vi "FPGAcode_6_02_14.vi"() -> ()   [LabVIEW 2013]
uses:
  <vilib>/Platform/TimedLoop/XDataNode/timing_clust.ctl
  <vilib>/Platform/TimedLoop/XDataNode/nitl_modes.ctl
  <vilib>/Platform/TimedLoop/XDataNode/wakeup.ctl
  <vilib>/rvi/Emulation/niFpgaSctlEmulationGetInTimedLoop.vi
  <vilib>/rvi/Emulation/niFpgaEmulationReportErrorSimple.vi
  <vilib>/rvi/Emulation/niFpgaGetClockAttributes.vi
  <vilib>/rvi/Emulation/niFpgaCriticalErrorInLSC.vi
  <vilib>/rvi/eio/common/nirviEmuTemplateMethod_errors.vi
  <vilib>/Platform/TimedLoop/XDataNode/XDataNode.xnode
  <vilib>/eio/EIONode/EIONode.xnode
  <vilib>/Platform/TimedLoop/XDataNode/XDNodeRunTimeDep.lvlib
panel:
  out "Not Armed?":bool
  in  "Reset One Shot":bool
  in  "One Shot":bool
  in  "Mult1 Use":bool
  out "Filter 1 Detector 3 Correlation":i32
  in  "Filter 2 threshold":i32=1000
  out "Filter 2 Detector 3 Correlation":i32
  in  "Filter 1 threshold":i32=1000
  in  "Filter 3 threshold":i32=1000
  out "Filter 3 Detector 3 Correlation":i32
  in  "Filter 4 threshold":i32=1000
  out "Filter 4 Detector 3 Correlation":i32
  in  "Filter 5 threshold":i32
  out "Filter 5 Detector 3 Correlation":i32
  in  "Filter 6 threshold":i32
  out "Filter 6 Detector 3 Correlation":i32
  in  "Filter 7 threshold":i32
  out "Filter 7 Detector 3 Correlation":i32
  out "Plates":bool
  in  "High Charge Limit":i16
  in  "Low Charge Limit":i16
  in  "High Velocity Count":i32
  in  "Low Velocity Count":i32
  in  "High Mass Limit":i64
  in  "Low Mass Limit":i64
  in  "Mult1":fxp<+,16,7>
  out "Delay1":bool
  out "IO Module\\AI 0":i16
  out "IO Module\\AI 1":i16
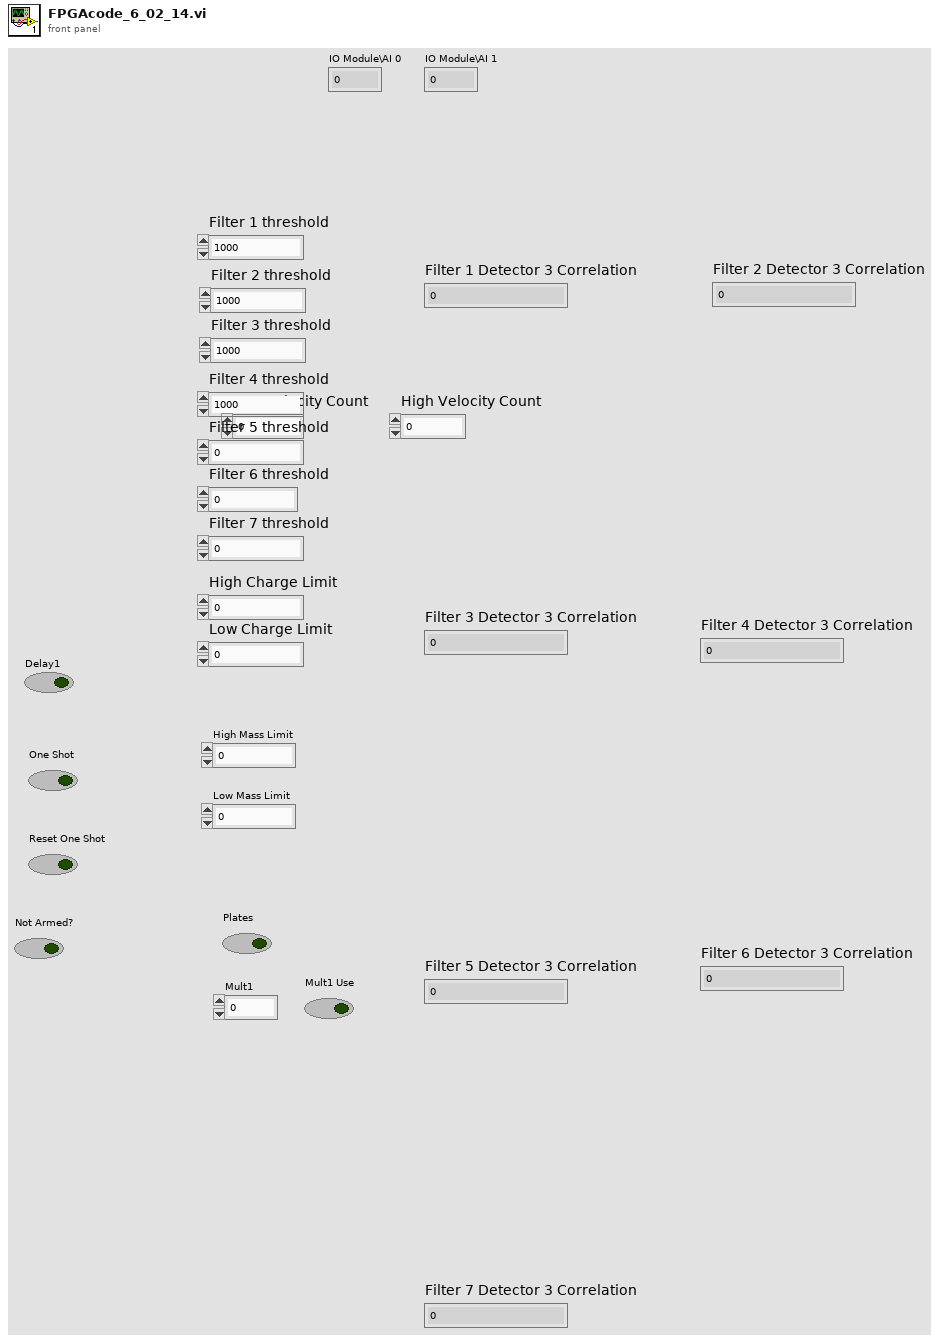
[diagram p1: front panel]
types:
  T1 = typedef "XDNodeRunTimeDep.lvlib/timing_clust.ctl" = cluster{"Expected End [f-1]":u64, "Actual End [f-1]":u64, "Finished Late? [f-1]":bool, "Expected End [i-1]":u64, "Actual End [i-1]":u64, "Finished Late? [i-1]":bool, "Expected Start [i]":u64, "Actual Start [i]":u64, "Expected Start [f]":u64, "Actual Start [f]":u64, "Source Name":string, "Structure Name":string, "Period":i64, "Deadline":i64, "Offset":i64, "Start":i64, "Priority":i32, "Timeout":i32, "Mode":T2, "Wakeup Reason":T3, "Error":errorcluster, "Source Type":string, "Secondary Source Type":string, "Global End Time":u64, "Global Start Time":u64, "Frame Duration":u64, "Iteration Duration":u64, "Assigned CPU":i32, "I/O Scan Engine Mode":u32}
  T2 = typedef "XDNodeRunTimeDep.lvlib/nitl_modes.ctl" = enum32{"No Change", "Process missed periods, maintain original phase", "Discard missed periods, maintain original phase", "Process missed periods, ignore original phase", "Discard missed periods, ignore original phase"}
  T3 = typedef "XDNodeRunTimeDep.lvlib/wakeup.ctl" = enum32{"Normal", "Aborted", "Asynchronous wakeup", "Timing source error", "Timed loop error", "Timeout"}
  T4 = cluster{"Separation cut off 1":i32, "Filter Number":i32, "Separation cut off 2":i32}
  T5 = cluster{"Old Average":i32, "New Average":i32, "Current State":u8, "Detector 1 Correlation":i32, "Detector 3 Correlation":i32, "Velocity Count":i32, "Detector Counter in":i32, "Timeout Count in":i32, "Measured Charge in":i32, "Filter Threshold":i32, "High Correlation in":i32, "Offset":i32, "Offset Average":i32, "Measured Velocity In":i32, "Mult Cluster":cluster{"Mult1":fxp<+,16,7>, "Mult1 Use?":bool}, "Final Delay Count In":u16, "Delay1 In":i32}
  T6 = cluster{"High Charge Limit":i16, "Low Charge Limit":i16, "Low Velocity Count":i32, "High Velocity Count":i32, "Low Velocity Count":i32, fxp<+,30,25>, "High Mass Limit":i64, "Low Mass Limit":i64}
  T7 = cluster{"Average Out":i32, "Next State":u8, "Velocity Count out":i32, "Detector counter out":i32, "Timeout count out":u32, "Measured Charge Out":i32, "High Correlation Out":i32, "Plates":bool, "Offset Out":i32, "Measured Velocity Out":i32, "Final Delay Count Out":u16, "Out1":bool, "Delay1":i32}
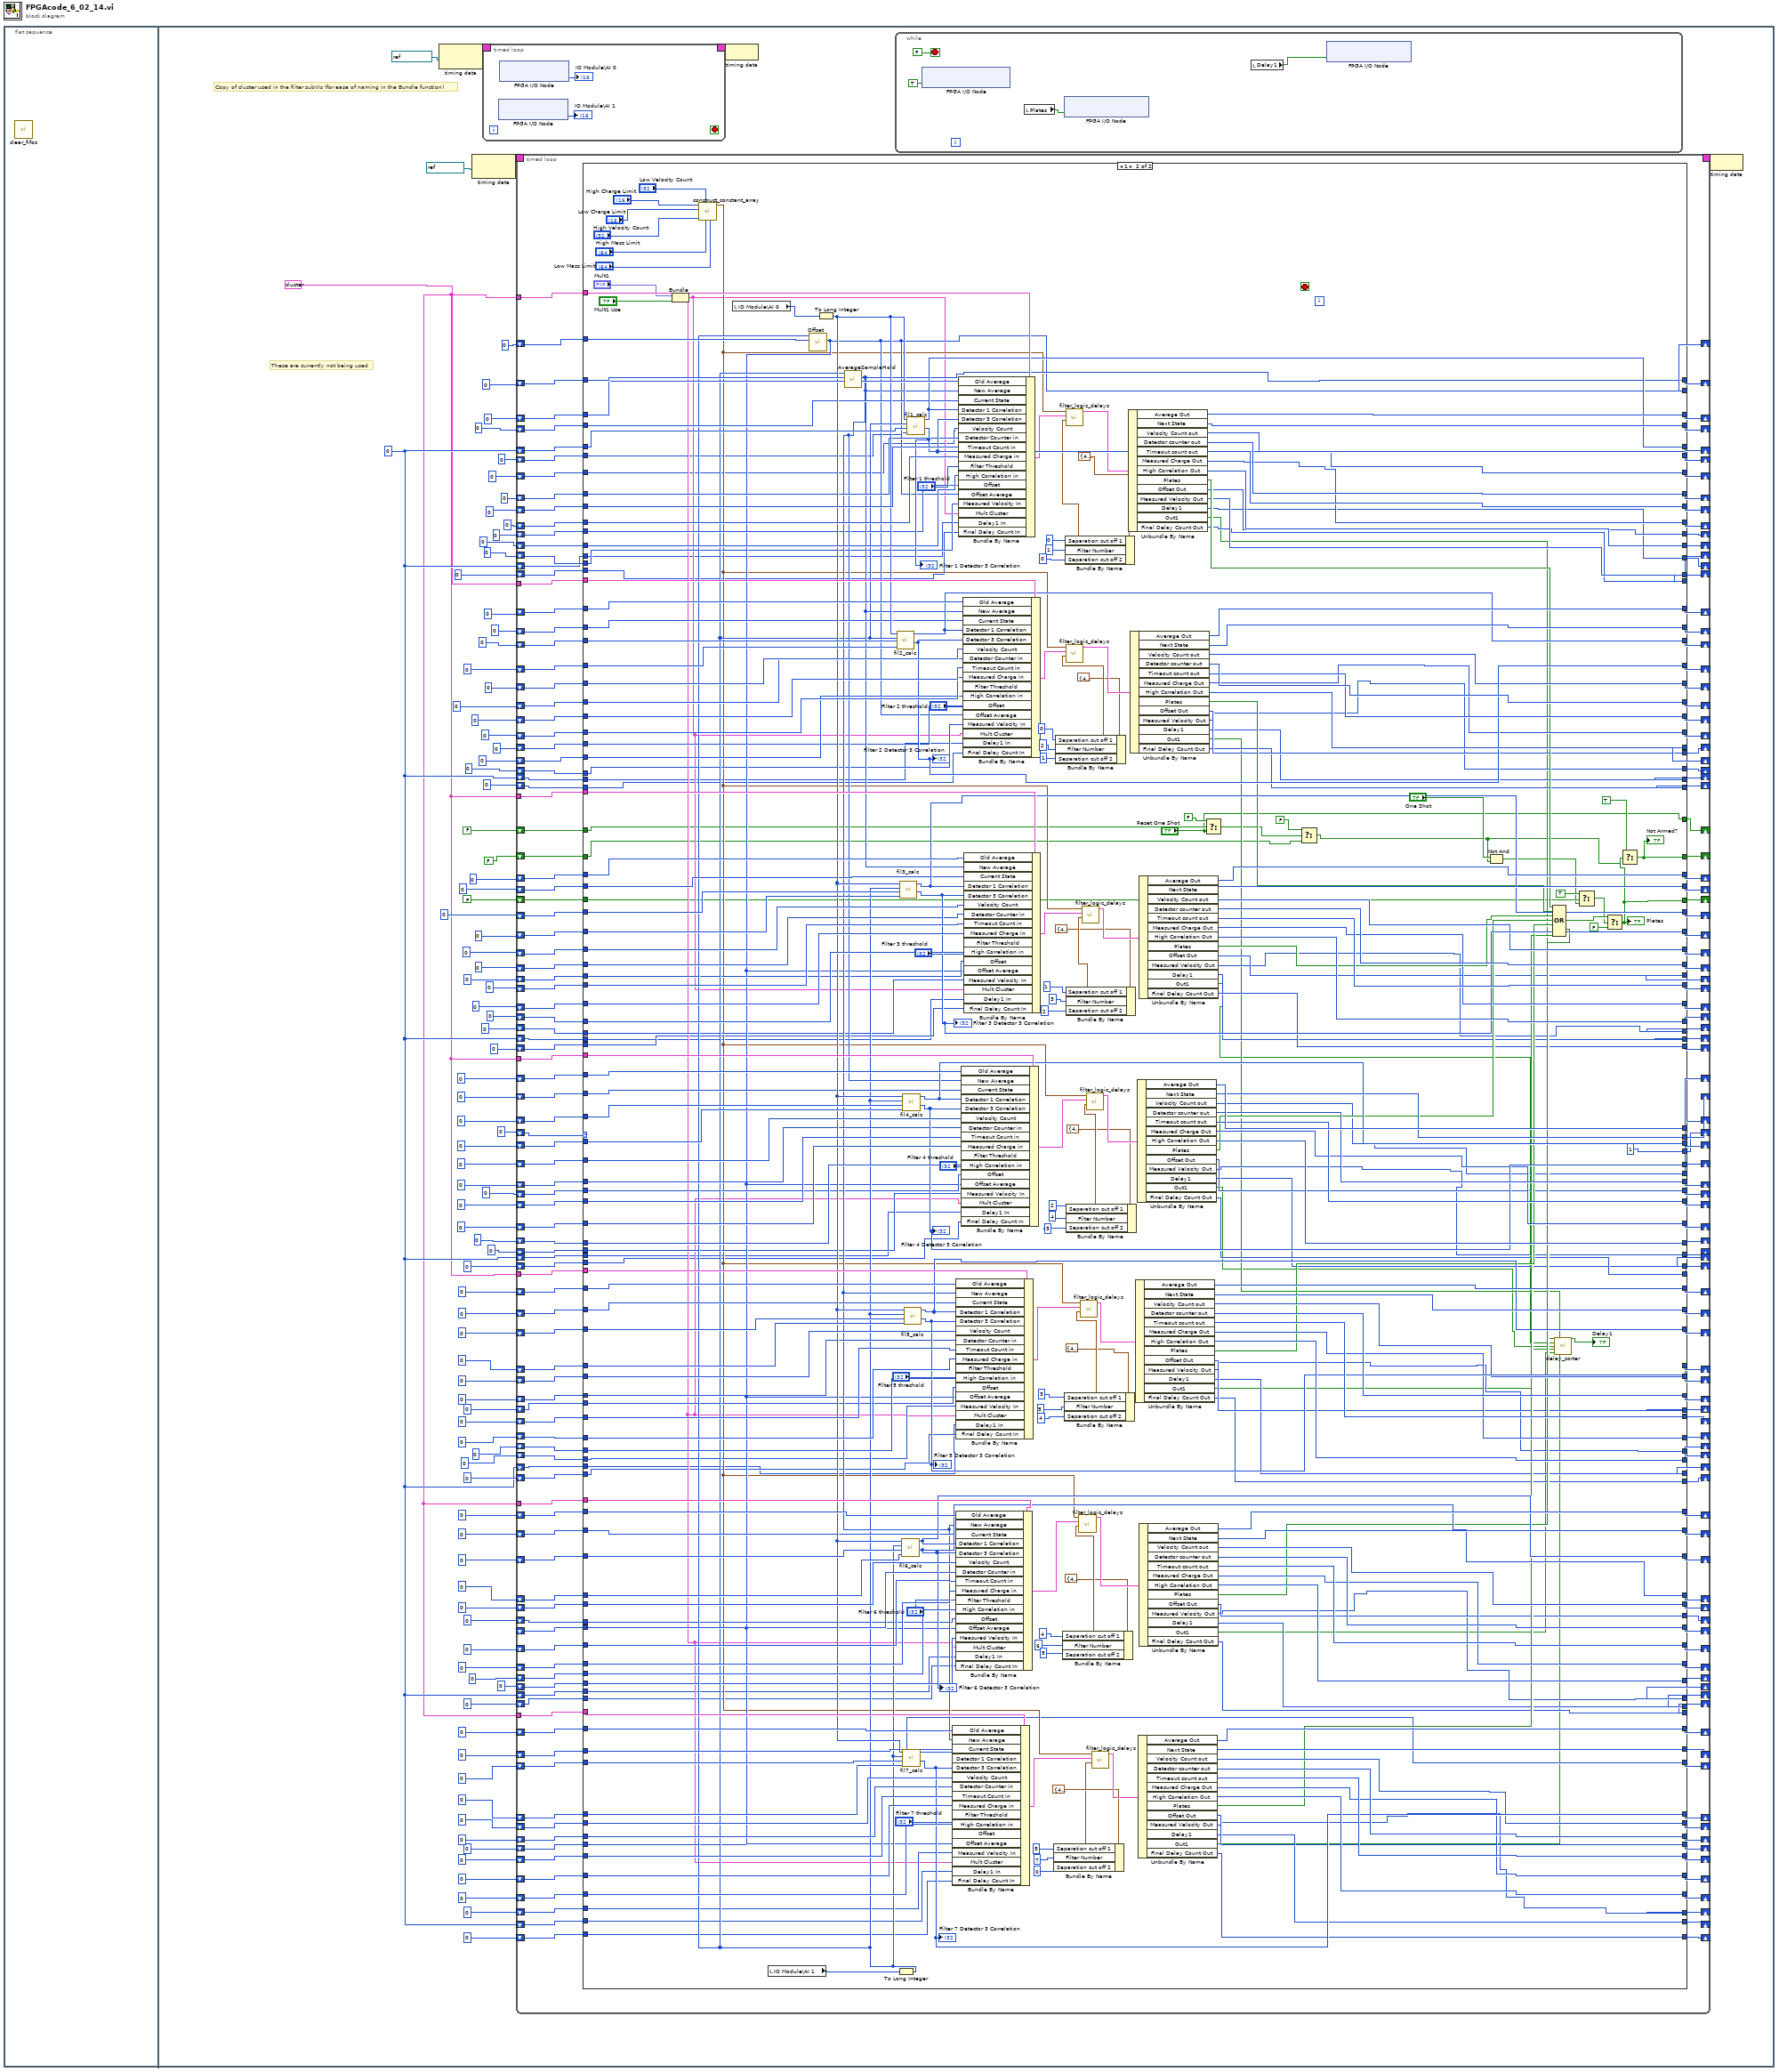
[diagram p0: block diagram]
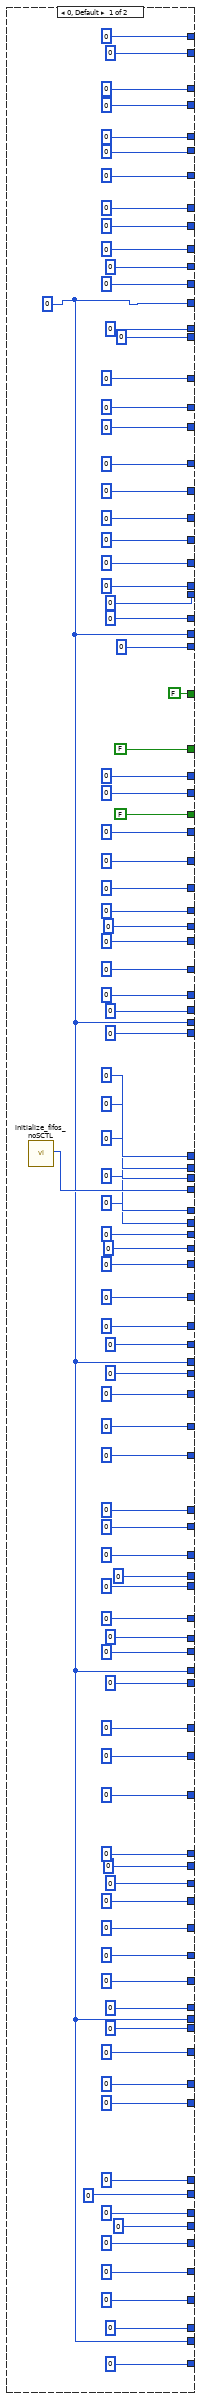
[diagram p2: hidden frame]
diagram:
  n1 = flat-sequence {
    frame #0 {
      n2 = call "clear_fifos.vi"() -> ()  [unwired: 1 in]
    }
    frame #1 {
      w2 = T5 {"Old Average"=0, "New Average"=0, "Current State"=0, "Detector 1 Correlation"=0, "Detector 3 Correlation"=0, "Velocity Count"=0, "Detector Counter in"=0, "Timeout Count in"=0, "Measured Charge in"=0, "Filter Threshold"=0, "High Correlation in"=0, "Offset"=0, "Offset Average"=0, "Measured Velocity In"=0, "Mult Cluster"={"Mult1"=0.0, "Mult1 Use?"=FALSE}, "Final Delay Count In"=0, "Delay1 In"=0} ("Variables Cluster")
      w5 = 0 ("Detector 1 Correlation Out")
      # "These are currently not being used"
      # "Copy of cluster used in the filter subVIs (for ease of naming in the Bundle function)"
      n3 = node-c288(refnum<k21> "AI Clock" ("Source Name")) -> (w32:T1)
      n4 = node-c288(refnum<k21> "26 MHz" ("Source Name")) -> (w96:T1)
      n5 = timed-loop {
        timing: w32 -> [_]
        timing-out: [_] -> w31
        stop <- _ stop-if-true
        n6 = xnode "FPGA I/O Node"() -> ("IO Module\\AI 1"=→"IO Module\\AI 1":i16)  [unwired: 1 in, 1 out]
        n7 = xnode "FPGA I/O Node"() -> ("IO Module\\AI 0"=→"IO Module\\AI 0":i16)  [unwired: 1 in, 1 out]
      }
      n8 = timed-loop {
        timing: w96 -> [_]
        timing-out: [_] -> w95
        shift-right: [w302] -> _
        shift-left: 0 ("Velocity Count out") -> [w224]
        shift-right: [w303] -> _
        shift-left: 0 ("Detector 1 Correlation out") -> [w225]
        shift-right: [w189] -> _
        shift-left: 0 ("Detector counter out") -> [w226]
        shift-right: [w220] -> _
        shift-left: 0 ("Next State") -> [w227]
        shift-right: [w188] -> _
        shift-left: 0 ("Detector 3 Correlation out") -> [w223]
        shift-right: [w301] -> _
        shift-left: 0 ("Timeout count out") -> [w222]
        shift-right: [w216] -> _
        shift-left: 0 ("Next State") -> [w219]
        shift-right: [w215] -> _
        shift-left: 0 ("Detector counter out") -> [w218]
        shift-right: [w187] -> _
        shift-left: 0 ("Detector 1 Correlation out") -> [w295]
        shift-right: [w292] -> _
        shift-left: 0 ("Velocity Count out") -> [w294]
        shift-right: [w291] -> _
        shift-left: u32 0 ("Detector 3 Correlation out") -> [w293]
        shift-right: [w286] -> _
        shift-left: 0 ("Timeout count out") -> [w287]
        shift-right: [w210] -> _
        shift-left: 0 ("Next State") -> [w213]
        shift-right: [w185] -> _
        shift-left: 0 ("Detector counter out") -> [w283]
        shift-right: [w281] -> _
        shift-left: 0 ("Detector 1 Correlation out") -> [w282]
        shift-right: [w279] -> _
        shift-left: u32 0 ("Velocity Count out") -> [w280]
        shift-right: [w184] -> _
        shift-left: 0 ("Detector 3 Correlation out") -> [w278]
        shift-right: [w277] -> _
        shift-left: 0 ("Timeout count out") -> [w212]
        shift-right: [w304] -> _
        shift-left: u8 0 ("High Correlation Out") -> [w307]
        shift-right: [w296] -> _
        shift-left: u8 0 ("High Correlation Out") -> [w297]
        shift-right: [w211] -> _
        shift-left: 0 ("High Correlation Out") -> [w214]
        shift-right: [w305] -> _
        shift-left: 0 ("Measured Charge Out") -> [w308]
        shift-right: [w298] -> _
        shift-left: 0 ("Measured Charge Out") -> [w299]
        shift-right: [w285] -> _
        shift-left: u8 0 ("Measured Charge Out") -> [w284]
        shift-right: [w175] -> _
        shift-left: 0 ("Output New Average") -> [w309]
        shift-right: [w221] -> _
        shift-left: w5 -> [w228]
        tunnel: w2 -> [w306]
        shift-right: [w186] -> _
        shift-left: 0 ("High Sample Out") -> [w289]
        shift-right: [w290] -> _
        shift-left: 0 ("High Correlation Out") -> [w217]
        tunnel: w2 -> [w300]
        tunnel: w2 -> [w288]
        shift-right: [w276] -> _
        shift-left: 0 ("Average Out") -> [w275]
        shift-right: [w274] -> _
        shift-left: u8 0 ("Next State") -> [w273]
        shift-right: [w206] -> _
        shift-left: 0 ("Detector 1 Correlation out") -> [w208]
        shift-right: [w205] -> _
        shift-left: 0 ("Detector 3 Correlation out") -> [w207]
        shift-right: [w183] -> _
        shift-left: 0 ("Velocity Count out") -> [w272]
        shift-right: [w271] -> _
        shift-left: 0 ("Detector counter out") -> [w270]
        shift-right: [w269] -> _
        shift-left: u32 0 ("Timeout count out") -> [w268]
        shift-right: [w182] -> _
        shift-left: 0 ("Measured Charge Out") -> [w267]
        shift-right: [w266] -> _
        shift-left: 0 ("High Correlation Out") -> [w209]
        tunnel: w2 -> [w265]
        shift-right: [w263] -> _
        shift-left: 0 ("Average Out") -> [w262]
        shift-right: [w261] -> _
        shift-left: u8 0 ("Next State") -> [w260]
        shift-right: [w201] -> _
        shift-left: 0 ("Detector 1 Correlation out") -> [w204]
        shift-right: [w200] -> _
        shift-left: 0 ("Detector 3 Correlation out") -> [w203]
        shift-right: [w181] -> _
        shift-left: 0 ("Velocity Count out") -> [w259]
        shift-right: [w258] -> _
        shift-left: 0 ("Detector counter out") -> [w257]
        shift-right: [w256] -> _
        shift-left: u32 0 ("Timeout count out") -> [w255]
        shift-right: [w180] -> _
        shift-left: 0 ("Measured Charge Out") -> [w254]
        shift-right: [w253] -> _
        shift-left: 0 ("High Correlation Out") -> [w202]
        tunnel: w2 -> [w264]
        shift-right: [w251] -> _
        shift-left: 0 ("Average Out") -> [w249]
        shift-right: [w250] -> _
        shift-left: u8 0 ("Next State") -> [w246]
        shift-right: [w196] -> _
        shift-left: 0 ("Detector 1 Correlation out") -> [w199]
        shift-right: [w195] -> _
        shift-left: 0 ("Detector 3 Correlation out") -> [w198]
        shift-right: [w178] -> _
        shift-left: 0 ("Velocity Count out") -> [w248]
        shift-right: [w245] -> _
        shift-left: _ -> [w247]
        shift-right: [w244] -> _
        shift-left: u32 0 ("Timeout count out") -> [w243]
        shift-right: [w179] -> _
        shift-left: 0 ("Measured Charge Out") -> [w242]
        shift-right: [w241] -> _
        shift-left: 0 ("High Correlation Out") -> [w197]
        tunnel: w2 -> [w252]
        shift-right: [w239] -> _
        shift-left: 0 ("Average Out") -> [w238]
        shift-right: [w237] -> _
        shift-left: u8 0 ("Next State") -> [w229]
        shift-right: [w191] -> _
        shift-left: 0 ("Detector 1 Correlation out") -> [w194]
        shift-right: [w190] -> _
        shift-left: 0 ("Detector 3 Correlation out") -> [w193]
        shift-right: [w177] -> _
        shift-left: 0 ("Velocity Count out") -> [w236]
        shift-right: [w235] -> _
        shift-left: 0 ("Detector counter out") -> [w234]
        shift-right: [w233] -> _
        shift-left: u32 0 ("Timeout count out") -> [w232]
        shift-right: [w176] -> _
        shift-left: 0 ("Measured Charge Out") -> [w231]
        shift-right: [w230] -> _
        shift-left: 0 ("High Correlation Out") -> [w192]
        tunnel: w2 -> [w240]
        shift-right: [w173] -> _
        shift-left: i16 0 -> [w174]
        shift-right: [w171] -> _
        shift-left: 0 -> [w172]
        shift-right: [w170] -> _
        shift-left: 0 -> [w167]
        shift-right: [w168] -> _
        shift-left: 0 -> [w169]
        shift-right: [w165] -> _
        shift-left: 0 ("Offset Out") -> [w166]
        shift-right: [w164] -> _
        shift-left: 0 ("Offset Out") -> [w163]
        shift-right: [w162] -> _
        shift-left: 0 ("Offset Out") -> [w161]
        shift-right: [w160] -> _
        shift-left: 0 ("Offset Out") -> [w159]
        shift-right: [w158] -> _
        shift-left: 0 ("Offset Out") -> [w157]
        shift-right: [w155] -> _
        shift-left: 0 -> [w156]
        shift-right: [w154] -> _
        shift-left: 0 -> [w143]
        shift-right: [w153] -> _
        shift-left: 0 -> [w144]
        shift-right: [w152] -> _
        shift-left: 0 -> [w145]
        shift-right: [w151] -> _
        shift-left: 0 -> [w146]
        shift-right: [w150] -> _
        shift-left: 0 -> [w147]
        shift-right: [w149] -> _
        shift-left: 0 ("Measured Velocity Out") -> [w148]
        shift-right: [w142] -> _
        shift-left: w5 -> [w140]
        shift-right: [w141] -> _
        shift-left: u32 0 ("Final Delay Count Out") -> [w139]
        shift-right: [w138] -> _
        shift-left: w5 -> [w136]
        shift-right: [w137] -> _
        shift-left: u32 0 ("Final Delay Count Out") -> [w135]
        shift-right: [w134] -> _
        shift-left: w5 -> [w132]
        shift-right: [w133] -> _
        shift-left: u32 0 ("Final Delay Count Out") -> [w131]
        shift-right: [w130] -> _
        shift-left: w5 -> [w128]
        shift-right: [w129] -> _
        shift-left: u32 0 ("Final Delay Count Out") -> [w127]
        shift-right: [w126] -> _
        shift-left: w5 -> [w124]
        shift-right: [w125] -> _
        shift-left: u32 0 ("Final Delay Count Out") -> [w123]
        shift-right: [w122] -> _
        shift-left: w5 -> [w120]
        shift-right: [w121] -> _
        shift-left: u32 0 ("Final Delay Count Out") -> [w119]
        shift-right: [w118] -> _
        shift-left: w5 -> [w116]
        shift-right: [w117] -> _
        shift-left: u32 0 ("Final Delay Count Out") -> [w115]
        shift-right: [w113] -> _
        shift-left: FALSE -> [w114]
        shift-right: [w112] -> _
        shift-left: FALSE ("f") -> [w111]
        shift-right: [w110] -> _
        shift-left: FALSE ("Reset One Shot") -> [w109]
        stop <- _ stop-if-true
        n9 = case shown="1" w174 {
          tunnel: w309 -> [_ w696]
          tunnel: w308 -> [_ w695]
          tunnel: w307 -> [_ w530]
          tunnel: w306 -> [_ w694]
          tunnel: [0 ("Average Out") w693] -> w305
          tunnel: [u16 0 ("Next State") w692] -> w304
          tunnel: [0 ("Detector counter out") w691] -> w303
          tunnel: [u32 0 ("Timeout count out") w690] -> w302
          tunnel: [0 ("High Correlation Out") w689] -> w301
          tunnel: w300 -> [_ w688]
          tunnel: w299 -> [_ w687]
          tunnel: [0 ("Average Out") w686] -> w298
          tunnel: w297 -> [_ w529]
          tunnel: [u16 0 ("Next State") w685] -> w296
          tunnel: w295 -> [_ w684]
          tunnel: w294 -> [_ w522]
          tunnel: w293 -> [_ w683]
          tunnel: [0 ("Detector counter out") w682] -> w292
          tunnel: [u32 0 ("Timeout count out") w681] -> w291
          tunnel: [0 ("High Correlation Out") w680] -> w290
          tunnel: w289 -> [_ w679]
          tunnel: w288 -> [_ w678]
          tunnel: w287 -> [_ w677]
          tunnel: [0 ("Average Out") w676] -> w286
          tunnel: [u16 0 ("Next State") w675] -> w285
          tunnel: w284 -> [_ w528]
          tunnel: w283 -> [_ w674]
          tunnel: w282 -> [_ w521]
          tunnel: [0 ("Detector counter out") w673] -> w281
          tunnel: w280 -> [_ w672]
          tunnel: [u32 0 ("Timeout count out") w671] -> w279
          tunnel: w278 -> [_ w670]
          tunnel: [0 ("High Correlation Out") w669] -> w277
          tunnel: [0 ("Average Out") w668] -> w276
          tunnel: w275 -> [_ w667]
          tunnel: [u16 0 ("Next State") w666] -> w274
          tunnel: w273 -> [_ w527]
          tunnel: w272 -> [_ w665]
          tunnel: [0 ("Detector counter out") w664] -> w271
          tunnel: w270 -> [_ w520]
          tunnel: [u32 0 ("Timeout count out") w663] -> w269
          tunnel: w268 -> [_ w662]
          tunnel: w267 -> [_ w661]
          tunnel: [0 ("High Correlation Out") w660] -> w266
          tunnel: w265 -> [_ w659]
          tunnel: w264 -> [_ w658]
          tunnel: [0 ("Average Out") w657] -> w263
          tunnel: w262 -> [_ w656]
          tunnel: [u16 0 ("Next State") w655] -> w261
          tunnel: w260 -> [_ w526]
          tunnel: w259 -> [_ w654]
          tunnel: [0 ("Detector counter out") w653] -> w258
          tunnel: w257 -> [_ w519]
          tunnel: [u32 0 ("Timeout count out") w652] -> w256
          tunnel: w255 -> [_ w651]
          tunnel: w254 -> [_ w650]
          tunnel: [0 ("High Correlation Out") w649] -> w253
          tunnel: w252 -> [_ w648]
          tunnel: [0 ("Average Out") w647] -> w251
          tunnel: [u16 0 ("Next State") w646] -> w250
          tunnel: w249 -> [_ w645]
          tunnel: w248 -> [_ w644]
          tunnel: w247 -> [_ w518]
          tunnel: w246 -> [_ w525]
          tunnel: [0 ("Detector counter out") w643] -> w245
          tunnel: [u32 0 ("Timeout count out") w642] -> w244
          tunnel: w243 -> [_ w641]
          tunnel: w242 -> [_ w640]
          tunnel: [0 ("High Correlation Out") w639] -> w241
          tunnel: w240 -> [_ w638]
          tunnel: [0 ("Average Out") w637] -> w239
          tunnel: w238 -> [_ w636]
          tunnel: [u16 0 ("Next State") w635] -> w237
          tunnel: w236 -> [_ w634]
          tunnel: [0 ("Detector counter out") w633] -> w235
          tunnel: w234 -> [_ w517]
          tunnel: [u32 0 ("Timeout count out") w632] -> w233
          tunnel: w232 -> [_ w631]
          tunnel: w231 -> [_ w630]
          tunnel: [0 ("High Correlation Out") w629] -> w230
          tunnel: w229 -> [_ w524]
          tunnel: w228 -> [_ w628]
          tunnel: w227 -> [_ w423]
          tunnel: w226 -> [_ w424]
          tunnel: w225 -> [_ w523]
          tunnel: w224 -> [_ w627]
          tunnel: w223 -> [_ w626]
          tunnel: w222 -> [_ w625]
          tunnel: [0 ("Detector 1 Correlation Out") w624] -> w221
          tunnel: [0 ("Detector 3 Correlation Out") w623] -> w220
          tunnel: w219 -> [_ w622]
          tunnel: w218 -> [_ w621]
          tunnel: w217 -> [_ w620]
          tunnel: [0 ("Detector 1 Correlation Out") w619] -> w216
          tunnel: [0 ("Detector 3 Correlation Out") w618] -> w215
          tunnel: w214 -> [_ w617]
          tunnel: w213 -> [_ w616]
          tunnel: w212 -> [_ w615]
          tunnel: [0 ("Detector 1 Correlation Out") w614] -> w211
          tunnel: [0 ("Detector 3 Correlation Out") w613] -> w210
          tunnel: w209 -> [_ w612]
          tunnel: w208 -> [_ w611]
          tunnel: w207 -> [_ w610]
          tunnel: [0 ("Detector 1 Correlation Out") w609] -> w206
          tunnel: [0 ("Detector 3 Correlation Out") w608] -> w205
          tunnel: w204 -> [_ w607]
          tunnel: w203 -> [_ w606]
          tunnel: w202 -> [_ w605]
          tunnel: [0 ("Detector 1 Correlation Out") w604] -> w201
          tunnel: [0 ("Detector 3 Correlation Out") w603] -> w200
          tunnel: w199 -> [_ w602]
          tunnel: w198 -> [_ w601]
          tunnel: w197 -> [_ w600]
          tunnel: [0 ("Detector 1 Correlation Out") w599] -> w196
          tunnel: [0 ("Detector 3 Correlation Out") w598] -> w195
          tunnel: w194 -> [_ w597]
          tunnel: w193 -> [_ w596]
          tunnel: w192 -> [_ w595]
          tunnel: [0 ("Detector 1 Correlation Out") w460] -> w191
          tunnel: [0 ("Detector 3 Correlation Out") w594] -> w190
          tunnel: [0 ("Velocity Count out") w593] -> w189
          tunnel: [0 ("Measured Charge Out") w592] -> w188
          tunnel: [0 ("Velocity Count out") w591] -> w187
          tunnel: [0 ("Measured Charge Out") w590] -> w186
          tunnel: [0 ("Velocity Count out") w589] -> w185
          tunnel: [0 ("Measured Charge Out") w588] -> w184
          tunnel: [0 ("Velocity Count out") w516] -> w183
          tunnel: [0 ("Measured Charge Out") w587] -> w182
          tunnel: [0 ("Velocity Count out") w586] -> w181
          tunnel: [0 ("Measured Charge Out") w585] -> w180
          tunnel: [0 ("Measured Charge Out") w584] -> w179
          tunnel: [0 ("Velocity Count out") w583] -> w178
          tunnel: [0 ("Velocity Count out") w582] -> w177
          tunnel: [0 ("Measured Charge Out") w581] -> w176
          tunnel: [0 ("Output New Average") w515] -> w175
          tunnel: [w400 i16 1 ("Output State")] -> w173
          tunnel: w172 -> [_ w512]
          tunnel: [0 ("Offset Out") w511] -> w171
          tunnel: [0 ("Offset Out") w510] -> w170
          tunnel: w169 -> [_ w509]
          tunnel: [0 ("Output New Average") w498] -> w168
          tunnel: w167 -> [_ w507]
          tunnel: w166 -> [_ w506]
          tunnel: [0 ("Offset Out") w505] -> w165
          tunnel: [0 ("Offset Out") w504] -> w164
          tunnel: w163 -> [_ w503]
          tunnel: [0 ("Offset Out") w502] -> w162
          tunnel: w161 -> [_ w501]
          tunnel: [0 ("Offset Out") w500] -> w160
          tunnel: w159 -> [_ w499]
          tunnel: [0 ("Offset Out") w497] -> w158
          tunnel: w157 -> [_ w496]
          tunnel: w156 -> [_ w491]
          tunnel: [0 ("Measured Velocity Out") w484] -> w155
          tunnel: [0 ("Measured Velocity Out") w483] -> w154
          tunnel: [0 ("Measured Velocity Out") w482] -> w153
          tunnel: [0 ("Measured Velocity Out") w481] -> w152
          tunnel: [0 ("Measured Velocity Out") w480] -> w151
          tunnel: [0 ("Measured Velocity Out") w479] -> w150
          tunnel: [0 ("Measured Velocity Out") w478] -> w149
          tunnel: w148 -> [_ w490]
          tunnel: w147 -> [_ w489]
          tunnel: w146 -> [_ w488]
          tunnel: w145 -> [_ w487]
          tunnel: w144 -> [_ w486]
          tunnel: w143 -> [_ w485]
          tunnel: [w313 w455] -> w142
          tunnel: [u32 0 ("Final Delay Count Out") w473] -> w141
          tunnel: w140 -> [_ w472]
          tunnel: w139 -> [_ w471]
          tunnel: [w313 w470] -> w138
          tunnel: [u32 0 ("Final Delay Count Out") w469] -> w137
          tunnel: w136 -> [_ w468]
          tunnel: w135 -> [_ w467]
          tunnel: [w313 w453] -> w134
          tunnel: [u32 0 ("Final Delay Count Out") w466] -> w133
          tunnel: w132 -> [_ w446]
          tunnel: w131 -> [_ w465]
          tunnel: [w313 w452] -> w130
          tunnel: [u32 0 ("Final Delay Count Out") w464] -> w129
          tunnel: w128 -> [_ w445]
          tunnel: w127 -> [_ w463]
          tunnel: [w313 w451] -> w126
          tunnel: [u32 0 ("Final Delay Count Out") w462] -> w125
          tunnel: w124 -> [_ w444]
          tunnel: w123 -> [_ w461]
          tunnel: [w313 w450] -> w122
          tunnel: [u32 0 ("Final Delay Count Out") w459] -> w121
          tunnel: w120 -> [_ w443]
          tunnel: w119 -> [_ w458]
          tunnel: [w313 w449] -> w118
          tunnel: [u32 0 ("Final Delay Count Out") w457] -> w117
          tunnel: w116 -> [_ w442]
          tunnel: w115 -> [_ w456]
          tunnel: w114 -> [_ w408]
          tunnel: [FALSE ("t") w406] -> w113
          tunnel: [FALSE ("f") w420] -> w112
          tunnel: w111 -> [_ w419]
          tunnel: [FALSE ("Reset One Shot") "Reset One Shot"] -> w110
          tunnel: w109 -> [_ w404]
          frame 0, Default {
            w313 = 0
            n10 = call "initialize_fifos_noSCTL.vi"() -> ("Output State"=w400:i16)  [unwired: 11 in]
          }
          frame 1 {
            n11 = Bundle("Mult1"="Mult1", "Mult1 Use"="Mult1 Use") -> (w474:cluster{"Mult1":fxp<+,16,7>, "Mult1 Use":bool})  [unwired: 1 in]
            n12 = call "construct_constant_array.vi"("Low Mass Limit"="Low Mass Limit", "High Mass Limit"="High Mass Limit", "Low Velocity Count"="Low Velocity Count", "High Velocity Count"="High Velocity Count", "Low Charge Limit"="Low Charge Limit", "High Charge Limit"="High Charge Limit") -> ("constants cluster"=w475:T6)  [unwired: 5 in]
            n13 = local read "IO Module\\AI 0"() -> (w514:i16)
            n14 = local read "IO Module\\AI 1"() -> (w513:i16)
            n15 = To Long Integer(number=w514) -> (32bit integer=w539:i32)
            n16 = To Long Integer(number=w513) -> (32bit integer=w508:i32)
            n17 = call "Offset.vi"("Previous Average"=w509, "Input Value"=w508) -> ("Output New Average"=w498:i32)  [unwired: 7 in]
            n18 = call "AverageSampleHold.vi"("Previous Average"=w696, "Input Value"=w508) -> ("Output New Average"=w515:i32)  [unwired: 7 in]
            n19 = call "fil2_calc.vi"("Detector 3 Correlation In"=w621, "Detector 1 Correlation In"=w622, "AI1"=w508, "AI0"=w539) -> ("Detector 3 Correlation Out"=w618:i32, "Detector 1 Correlation Out"=w619:i32)  [unwired: 4 in]
            "Filter 2 Detector 3 Correlation" <- w618
            n20 = call "fil3_calc.vi"("Detector 3 Correlation In"=w616, "Detector 1 Correlation In"=w617, "AI1"=w508, "AI0"=w539) -> ("Detector 3 Correlation Out"=w613:i32, "Detector 1 Correlation Out"=w614:i32)  [unwired: 4 in]
            "Filter 3 Detector 3 Correlation" <- w613
            n21 = call "fil6_calc.vi"("Detector 3 Correlation In"=w601, "Detector 1 Correlation In"=w602, "AI1"=w508, "AI0"=w539) -> ("Detector 3 Correlation Out"=w598:i32, "Detector 1 Correlation Out"=w599:i32)  [unwired: 4 in]
            "Filter 6 Detector 3 Correlation" <- w598
            n22 = call "fil4_calc.vi"("Detector 3 Correlation In"=w610, "Detector 1 Correlation In"=w611, "AI1"=w508, "AI0"=w539) -> ("Detector 3 Correlation Out"=w608:i32, "Detector 1 Correlation Out"=w609:i32)  [unwired: 4 in]
            "Filter 4 Detector 3 Correlation" <- w608
            n23 = call "fil7_calc.vi"("Detector 3 Correlation In"=w596, "Detector 1 Correlation In"=w597, "AI1"=w508, "AI0"=w539) -> ("Detector 3 Correlation Out"=w594:i32, "Detector 1 Correlation Out"=w460:i32)  [unwired: 4 in]
            "Filter 7 Detector 3 Correlation" <- w594
            n24 = call "fil5_calc.vi"("Detector 3 Correlation In"=w606, "Detector 1 Correlation In"=w607, "AI1"=w508, "AI0"=w539) -> ("Detector 3 Correlation Out"=w603:i32, "Detector 1 Correlation Out"=w604:i32)  [unwired: 4 in]
            "Filter 5 Detector 3 Correlation" <- w603
            n25 = call "fil1_calc.vi"("Detector 3 Correlation In"=w423, "Detector 1 Correlation In"=w628, "AI1"=w508, "AI0"=w539) -> ("Detector 3 Correlation Out"=w623:i32, "Detector 1 Correlation Out"=w624:i32)  [unwired: 4 in]
            "Filter 1 Detector 3 Correlation" <- w623
            n26 = Bundle By Name(cluster=w638, "Old Average"=w636, "New Average"=w515, "Current State"=w524, "Detector 1 Correlation"=w460, "Detector 3 Correlation"=w594, "Velocity Count"=w634, "Detector Counter in"=w517, "Timeout Count in"=w631, "Measured Charge in"=w630, "Filter Threshold"="Filter 7 threshold", "High Correlation in"=w595, "Offset"=w496, "Offset Average"=w498, "Measured Velocity In"=w490, "Mult Cluster"=w474, "Delay1 In"=w442, "Final Delay Count In"=w456) -> (w409:T5)
            n27 = Bundle By Name(cluster=w648, "Old Average"=w645, "New Average"=w515, "Current State"=w525, "Detector 1 Correlation"=w599, "Detector 3 Correlation"=w598, "Velocity Count"=w644, "Detector Counter in"=w518, "Timeout Count in"=w641, "Measured Charge in"=w640, "Filter Threshold"="Filter 6 threshold", "High Correlation in"=w600, "Offset"=w499, "Offset Average"=w498, "Measured Velocity In"=w489, "Mult Cluster"=w474, "Delay1 In"=w443, "Final Delay Count In"=w458) -> (w410:T5)
            n28 = Bundle By Name(cluster=w658, "Old Average"=w656, "New Average"=w515, "Current State"=w526, "Detector 1 Correlation"=w604, "Detector 3 Correlation"=w603, "Velocity Count"=w654, "Detector Counter in"=w519, "Timeout Count in"=w651, "Measured Charge in"=w650, "Filter Threshold"="Filter 5 threshold", "High Correlation in"=w605, "Offset"=w501, "Offset Average"=w498, "Measured Velocity In"=w488, "Mult Cluster"=w474, "Delay1 In"=w444, "Final Delay Count In"=w461) -> (w411:T5)
            n29 = Bundle By Name(cluster=w694, "Old Average"=w695, "New Average"=w515, "Current State"=w530, "Detector 1 Correlation"=w624, "Detector 3 Correlation"=w623, "Velocity Count"=w424, "Detector Counter in"=w523, "Timeout Count in"=w627, "Measured Charge in"=w626, "Filter Threshold"="Filter 1 threshold", "High Correlation in"=w625, "Offset"=w512, "Offset Average"=w498, "Measured Velocity In"=w491, "Mult Cluster"=w474, "Delay1 In"=w472, "Final Delay Count In"=w471) -> (w415:T5)
            n30 = Bundle By Name(cluster=w659, "Old Average"=w667, "New Average"=w515, "Current State"=w527, "Detector 1 Correlation"=w609, "Detector 3 Correlation"=w608, "Velocity Count"=w665, "Detector Counter in"=w520, "Timeout Count in"=w662, "Measured Charge in"=w661, "Filter Threshold"="Filter 4 threshold", "High Correlation in"=w612, "Offset"=w503, "Offset Average"=w498, "Measured Velocity In"=w487, "Mult Cluster"=w474, "Delay1 In"=w445, "Final Delay Count In"=w463) -> (w412:T5)
            n31 = Bundle By Name(cluster=w688, "Old Average"=w687, "New Average"=w515, "Current State"=w529, "Detector 1 Correlation"=w619, "Detector 3 Correlation"=w618, "Velocity Count"=w684, "Detector Counter in"=w522, "Timeout Count in"=w683, "Measured Charge in"=w679, "Filter Threshold"="Filter 2 threshold", "High Correlation in"=w620, "Offset"=w507, "Offset Average"=w498, "Measured Velocity In"=w485, "Mult Cluster"=w474, "Delay1 In"=w468, "Final Delay Count In"=w467) -> (w414:T5)
            n32 = Bundle By Name(cluster=w678, "Old Average"=w677, "New Average"=w515, "Current State"=w528, "Detector 1 Correlation"=w614, "Detector 3 Correlation"=w613, "Velocity Count"=w674, "Detector Counter in"=w521, "Timeout Count in"=w672, "Measured Charge in"=w670, "Filter Threshold"="Filter 3 threshold", "High Correlation in"=w615, "Offset"=w506, "Offset Average"=w498, "Measured Velocity In"=w486, "Mult Cluster"=w474, "Delay1 In"=w446, "Final Delay Count In"=w465) -> (w413:T5)
            n33 = Bundle By Name(cluster=T4 {"Separation cut off 1"=4, "Filter Number"=5, "Separation cut off 2"=6} ("Filter Specific Constants"), "Separation cut off 1"=5, "Filter Number"=7, "Separation cut off 2"=0) -> (w427:T4)
            n34 = Bundle By Name(cluster=T4 {"Separation cut off 1"=4, "Filter Number"=5, "Separation cut off 2"=6} ("Filter Specific Constants"), "Separation cut off 1"=0, "Filter Number"=2, "Separation cut off 2"=1) -> (w572:T4)
            n35 = Bundle By Name(cluster=T4 {"Separation cut off 1"=4, "Filter Number"=5, "Separation cut off 2"=6} ("Filter Specific Constants"), "Separation cut off 1"=4, "Filter Number"=6, "Separation cut off 2"=5) -> (w562:T4)
            n36 = Bundle By Name(cluster=T4 {"Separation cut off 1"=4, "Filter Number"=5, "Separation cut off 2"=6} ("Filter Specific Constants"), "Separation cut off 1"=3, "Filter Number"=5, "Separation cut off 2"=4) -> (w564:T4)
            n37 = Bundle By Name(cluster=T4 {"Separation cut off 1"=4, "Filter Number"=5, "Separation cut off 2"=6} ("Filter Specific Constants"), "Separation cut off 1"=0, "Filter Number"=1, "Separation cut off 2"=0) -> (w570:T4)
            n38 = call "filter_logic_delays.vi"("Filter Specific Constants"=w570, "Variables Cluster"=w415, "controls cluster"=w475) -> ("Output Cluster"=w569:T7)  [unwired: 8 in]
            n39 = call "filter_logic_delays.vi"("Filter Specific Constants"=w572, "Variables Cluster"=w414, "controls cluster"=w475) -> ("Output Cluster"=w579:T7)  [unwired: 8 in]
            n40 = Bundle By Name(cluster=T4 {"Separation cut off 1"=4, "Filter Number"=5, "Separation cut off 2"=6} ("Filter Specific Constants"), "Separation cut off 1"=1, "Filter Number"=3, "Separation cut off 2"=2) -> (w568:T4)
            n41 = Bundle By Name(cluster=T4 {"Separation cut off 1"=4, "Filter Number"=5, "Separation cut off 2"=6} ("Filter Specific Constants"), "Separation cut off 1"=2, "Filter Number"=4, "Separation cut off 2"=3) -> (w566:T4)
            n42 = call "filter_logic_delays.vi"("Filter Specific Constants"=w562, "Variables Cluster"=w410, "controls cluster"=w475) -> ("Output Cluster"=w561:T7)  [unwired: 8 in]
            n43 = call "filter_logic_delays.vi"("Filter Specific Constants"=w564, "Variables Cluster"=w411, "controls cluster"=w475) -> ("Output Cluster"=w563:T7)  [unwired: 8 in]
            n44 = call "filter_logic_delays.vi"("Filter Specific Constants"=w568, "Variables Cluster"=w413, "controls cluster"=w475) -> ("Output Cluster"=w567:T7)  [unwired: 8 in]
            n45 = call "filter_logic_delays.vi"("Filter Specific Constants"=w566, "Variables Cluster"=w412, "controls cluster"=w475) -> ("Output Cluster"=w565:T7)  [unwired: 8 in]
            n46 = call "filter_logic_delays.vi"("Filter Specific Constants"=w427, "Variables Cluster"=w409, "controls cluster"=w475) -> ("Output Cluster"=w571:T7)  [unwired: 8 in]
            n47 = Unbundle By Name(w569) -> ("Average Out"=w693:i32, "Next State"=w692:u8, "Velocity Count out"=w593:i32, "Detector counter out"=w691:i32, "Timeout count out"=w690:u32, "Measured Charge Out"=w592:i32, "High Correlation Out"=w689:i32, "Plates"=w537:bool, "Offset Out"=w511:i32, "Measured Velocity Out"=w484:i32, "Delay1"=w455:i32, "Out1"=w448:bool, "Final Delay Count Out"=w473:u16)
            n48 = Unbundle By Name(w579) -> ("Average Out"=w686:i32, "Next State"=w685:u8, "Velocity Count out"=w591:i32, "Detector counter out"=w682:i32, "Timeout count out"=w681:u32, "Measured Charge Out"=w590:i32, "High Correlation Out"=w680:i32, "Plates"=w536:bool, "Offset Out"=w510:i32, "Measured Velocity Out"=w483:i32, "Delay1"=w470:i32, "Out1"=w447:bool, "Final Delay Count Out"=w469:u16)
            n49 = Unbundle By Name(w563) -> ("Average Out"=w657:i32, "Next State"=w655:u8, "Velocity Count out"=w586:i32, "Detector counter out"=w653:i32, "Timeout count out"=w652:u32, "Measured Charge Out"=w585:i32, "High Correlation Out"=w649:i32, "Plates"=w533:bool, "Offset Out"=w502:i32, "Measured Velocity Out"=w480:i32, "Delay1"=w451:i32, "Out1"=w437:bool, "Final Delay Count Out"=w462:u16)
            n50 = Unbundle By Name(w565) -> ("Average Out"=w668:i32, "Next State"=w666:u8, "Velocity Count out"=w516:i32, "Detector counter out"=w664:i32, "Timeout count out"=w663:u32, "Measured Charge Out"=w587:i32, "High Correlation Out"=w660:i32, "Plates"=w534:bool, "Offset Out"=w504:i32, "Measured Velocity Out"=w481:i32, "Delay1"=w452:i32, "Out1"=w438:bool, "Final Delay Count Out"=w464:u16)
            n51 = Unbundle By Name(w571) -> ("Average Out"=w637:i32, "Next State"=w635:u8, "Velocity Count out"=w582:i32, "Detector counter out"=w633:i32, "Timeout count out"=w632:u32, "Measured Charge Out"=w581:i32, "High Correlation Out"=w629:i32, "Plates"=w531:bool, "Offset Out"=w497:i32, "Measured Velocity Out"=w478:i32, "Delay1"=w449:i32, "Out1"=w436:bool, "Final Delay Count Out"=w457:u16)
            n52 = Unbundle By Name(w561) -> ("Average Out"=w647:i32, "Next State"=w646:u8, "Velocity Count out"=w583:i32, "Detector counter out"=w643:i32, "Timeout count out"=w642:u32, "Measured Charge Out"=w584:i32, "High Correlation Out"=w639:i32, "Plates"=w532:bool, "Offset Out"=w500:i32, "Measured Velocity Out"=w479:i32, "Delay1"=w450:i32, "Out1"=w435:bool, "Final Delay Count Out"=w459:u16)
            n53 = Unbundle By Name(w567) -> ("Average Out"=w676:i32, "Next State"=w675:u8, "Velocity Count out"=w589:i32, "Detector counter out"=w673:i32, "Timeout count out"=w671:u32, "Measured Charge Out"=w588:i32, "High Correlation Out"=w669:i32, "Plates"=w535:bool, "Offset Out"=w505:i32, "Measured Velocity Out"=w482:i32, "Delay1"=w453:i32, "Out1"=w439:bool, "Final Delay Count Out"=w466:u16)
            n54 = Select(t=FALSE, s=w404, f="Reset One Shot") -> (s? t:f=w402:bool)
            n55 = Select(t=FALSE, s=w402, f=w408) -> (s? t:f=w407:bool)
            n56 = Not And(1:w407, 2:"One Shot") -> (0:w417:bool)
            n57 = Compound Arithmetic op=OR(w537, w536, w535, w534, w533, w532, w531) -> (w426:bool)
            n58 = call "delay_sorter.vi"("Out1 1"=w448, "Out1 2"=w447, "Out1 3"=w439, "Out1 4"=w438, "Out1 5"=w437, "Out1 6"=w435, "Out1 7"=w436) -> ("Delay1"=→"Delay1":bool)  [unwired: 8 in]
            n59 = Select(t=TRUE, s=w419, f=w417) -> (s? t:f=w416:bool)
            n60 = Select(t=w426, s=w416, f=FALSE) -> (s? t:f=w420:bool)
            "Plates" <- w420
            n61 = Select(t=TRUE, s=w420, f=w407) -> (s? t:f=w406:bool)
            "Not Armed?" <- w406
          }
        }
      }
      n62 = node-c288(w31) -> ()
      n63 = while {
        stop <- FALSE stop-if-true
        n64 = xnode "FPGA I/O Node"("IO Module\\PFI Enable"=TRUE ("IO Module\\PFI Enable")) -> ()  [unwired: 1 in, 1 out]
        n65 = local read "Plates"() -> (w108:bool)
        n66 = xnode "FPGA I/O Node"("IO Module\\PFI Out 4"=w108) -> ()  [unwired: 1 in, 1 out]
        n67 = local read "Delay1"() -> (w105:bool)
        n68 = xnode "FPGA I/O Node"("IO Module\\PFI Out 1"=w105) -> ()  [unwired: 1 in, 1 out]
      }
      n69 = node-c288(w95) -> ()
    }
  }
